vi "Vergleicher.vi"(10 "Array":sgl[](array[numeric]), 11 "Numerisch":sgl) -> (1 "Änderung":bool)   [LabVIEW 2020, in "Allgemein.lvlib"]
uses:
  Allgemein.lvlib
panel:
  # "Ablaufinvariante Ausführung"
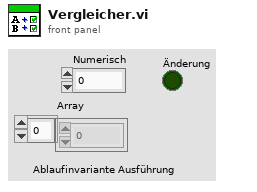
[diagram p1: front panel]
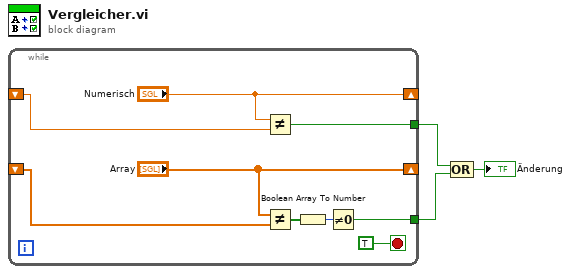
[diagram p0: block diagram]
diagram:
  n1 = while {
    shift-right: ["Numerisch"] -> _
    shift-left: _ -> [w9]
    tunnel: [w7] -> w2
    shift-right: ["Array"] -> _
    shift-left: _ -> [w6]
    tunnel: [w4] -> w3
    stop <- TRUE stop-if-true
    n2 = Not Equal?(x="Numerisch", y=w9) -> (x != y?=w7:bool)
    n3 = Not Equal?(x="Array", y=w6) -> (x != y?=w11:bool[])
    n4 = Boolean Array To Number(Boolean array=w11) -> (number=w10:u32)
    n5 = Not Equal To 0?(x=w10) -> (x != 0?=w4:bool)
  }
  n6 = Compound Arithmetic op=OR ("Mehrfacharithmetik")(w2, w3) -> (→"Änderung":bool)
